vi "IO Name to Enable Line.vi"(8 "error in (no error)":errorcluster, 10 "IO Name":string, 11 "sbRIO-9651 in":refnum<class "sbRIO-9651.lvclass">) -> (0 "error out":errorcluster, 2 "Enable Line":string, 3 "sbRIO-9651 out":refnum<class "sbRIO-9651.lvclass">)   [LabVIEW 2014, in "sbRIO-9651.lvclass"]
uses:
  sbRIO-9651.lvclass
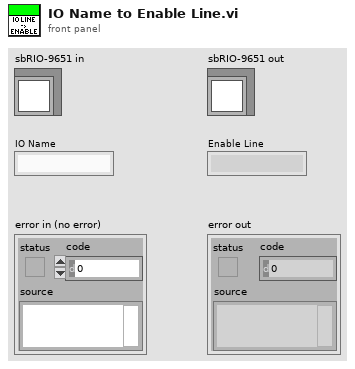
[diagram p1: front panel]
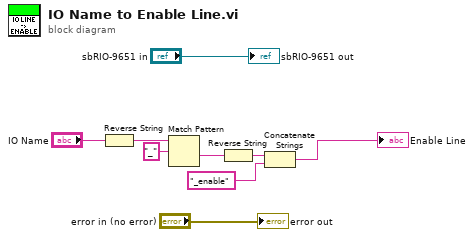
[diagram p0: block diagram]
diagram:
  n1 = Reverse String(1:"IO Name") -> (0:w6:string)
  n2 = Match Pattern(string=w6, regular expression="_") -> (after substring=w4:string)  [unwired: 1 in, 3 out]
  n3 = Reverse String(1:w4) -> (0:w3:string)
  n4 = Concatenate Strings(w3, "_enable" ("string")) -> (→"Enable Line":string)
  "error out" <- "error in (no error)"
  "sbRIO-9651 out" <- "sbRIO-9651 in"
